vi "Test_Send.vi"() -> ()   [LabVIEW 2020]
uses:
  <vilib>/Instr/_visa.llb/VISA Configure Serial Port (Serial Instr).vi
panel:
  out "INC":dbl min=0.0 max=12.0 step=0.1 format="%.1f"
  out "MPH":dbl min=0.0 max=12.0 step=0.1 format="%.1f"
  in  "Serial Port":refnum<visa-resource-name>="COM8"
  out "FootPath":path
  out "FootPathRef":refnum<file>
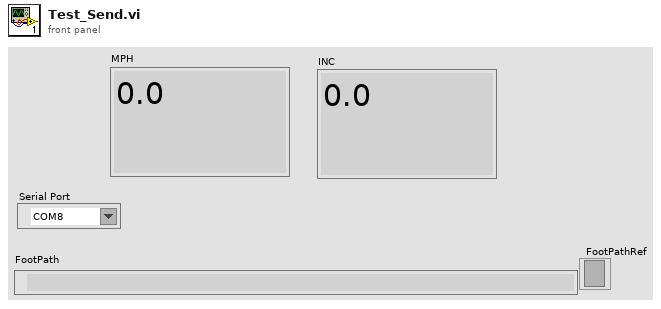
[diagram p1: front panel]
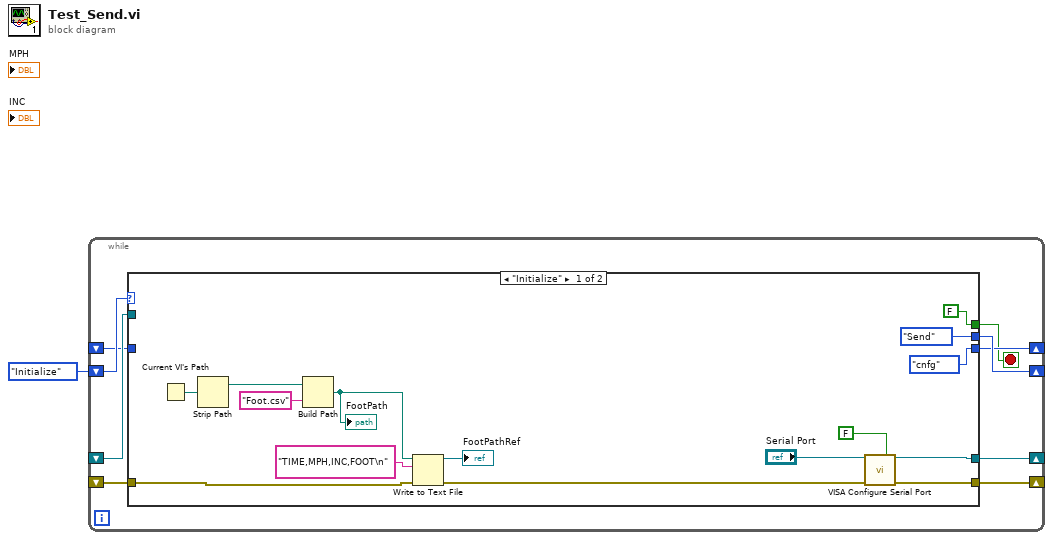
[diagram p0: block diagram]
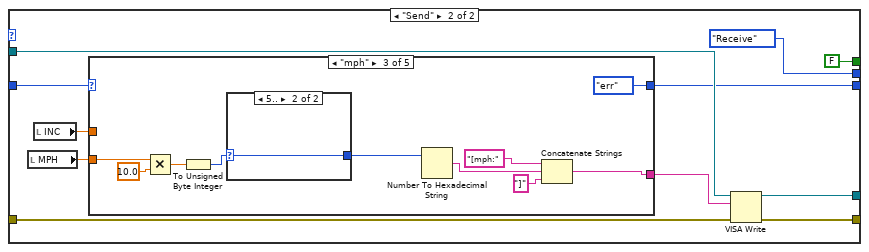
[diagram p2: hidden frame]
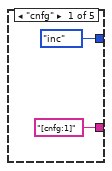
[diagram p3: hidden frame]
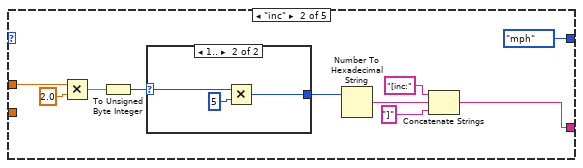
[diagram p4: hidden frame]
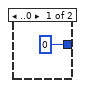
[diagram p5: hidden frame]
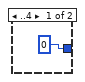
[diagram p6: hidden frame]
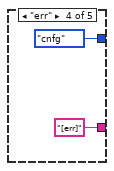
[diagram p7: hidden frame]
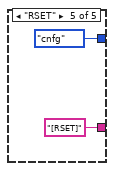
[diagram p8: hidden frame]
diagram:
  n1 = while {
    shift-right: [w6] -> _
    shift-left: _ -> [w10]
    shift-right: [w7] -> _
    shift-left: _ -> [w9]
    shift-right: [w5] -> _
    shift-left: enum16{"Initialize", "Send"}."Initialize" -> [w8]
    shift-right: [w4] -> _
    shift-left: _ -> [w3]
    stop <- w2 stop-if-true
    n2 = case shown="\"Initialize\"" w8 {
      tunnel: w10 -> [w13 w34]
      tunnel: w9 -> [_ w33]
      tunnel: [w23 w36] -> w7
      tunnel: [w22 w35] -> w6
      tunnel: [enum16{"Initialize", "Send"}."Send" enum16{"Initialize", "Send", "Receive", "Error"}."Receive"] -> w5
      tunnel: [enum16{"cnfg", "inc", "mph", "err", "RSET"}."cnfg" w30] -> w4
      tunnel: w3 -> [_ w31]
      tunnel: [FALSE FALSE] -> w2
      frame "Initialize" {
        n3 = Current VI's Path() -> (path=w18:path)
        n4 = Strip Path(path=w18) -> (stripped path=w17:path)  [unwired: 1 out]
        n5 = Build Path(base path=w17, name or relative path="Foot.csv") -> (appended path=w14:path)
        "FootPath" <- w14
        n6 = Write to Text File(file (use dialog)=w14, text="TIME,MPH,INC,FOOT\n", error in=w13) -> (refnum out=→"FootPathRef":refnum<file>, error out=w12:errorcluster)  [unwired: 1 in, 1 out]
        n7 = call-poly "VISA Configure Serial Port"("VISA resource name"="Serial Port", "Enable Termination\nChar (T)"=FALSE ("Enable Termination\nChar (T)"), "error in (no error)"=w12) -> ("VISA resource name out"=w23:refnum<visa-resource-name>, "error out"=w22:errorcluster)  [unwired: 11 in]
      }
      frame "Send" {
        n8 = local read "MPH"() -> (w27:dbl)
        n9 = local read "INC"() -> (w26:dbl)
        n10 = case shown="\"mph\"" w31 {
          tunnel: ["[cnfg:1]" w39 w53 "[err]" "[RSET]"] -> w32
          tunnel: w27 -> [_ _ w62 _ _]
          tunnel: [enum16{"cnfg", "inc", "mph", "err", "RSET"}."inc" enum16{"cnfg", "inc", "mph", "err", "RSET"}."mph" enum16{"cnfg", "inc", "mph", "err", "RSET"}."err" enum16{"cnfg", "inc", "mph", "err", "RSET"}."cnfg" enum16{"cnfg", "inc", "mph", "err", "RSET"}."cnfg"] -> w30
          tunnel: w26 -> [_ w40 _ _ _]
          frame "cnfg" {
          }
          frame "inc" {
            n11 = Multiply(x=w40, y=2.0) -> (x*y=w43:dbl)
            n12 = To Unsigned Byte Integer(number=w43) -> (unsigned 8bit integer=w42:u8)
            n13 = case shown="1.." w42 {
              selector: w42 -> [_ w52]
              tunnel: [u8 0 w51] -> w41
              frame ..0 {
              }
              frame 1.. {
                n14 = Multiply(x=w52, y=u8 5) -> (x*y=w51:u8)
              }
            }
            n15 = Number To Hexadecimal String(2:w41) -> (0:w46:string)  [unwired: 1 in]
            n16 = Concatenate Strings("[inc:" ("string"), w46, "]" ("string")) -> (w39:string)
          }
          frame "mph" {
            n17 = Multiply(x=w62, y=10.0) -> (x*y=w56:dbl)
            n18 = To Unsigned Byte Integer(number=w56) -> (unsigned 8bit integer=w55:u8)
            n19 = case shown="5.." w55 {
              selector: w55 -> [_ w64]
              tunnel: [u8 0 w64] -> w54
              frame ..4 {
              }
              frame 5.. {
              }
            }
            n20 = Number To Hexadecimal String(2:w54) -> (0:w59:string)  [unwired: 1 in]
            n21 = Concatenate Strings("[mph:" ("string"), w59, "]" ("string")) -> (w53:string)
          }
          frame "err" {
          }
          frame "RSET" {
          }
        }
        n22 = VISA Write(VISA resource name=w33, write buffer=w32, error in (no error)=w34) -> (VISA resource name out=w36:refnum<visa-resource-name>, error out=w35:errorcluster)  [unwired: 1 out]
      }
    }
  }
